vi "Create gplugindata payload.vi"(8 "error in":errorcluster, 9 "Library name with version":string, 10 "Relative Path":string, 11 "Display Name":string) -> (0 "error out":errorcluster, 3 "gplugindata":string)   [LabVIEW 2021, in "CIF Build Actions.lvlib"]
uses:
  CIF Build Actions.lvlib
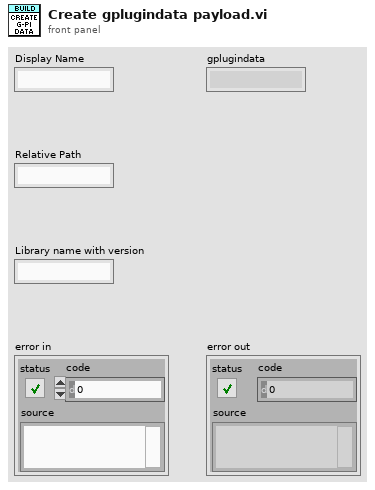
[diagram p1: front panel]
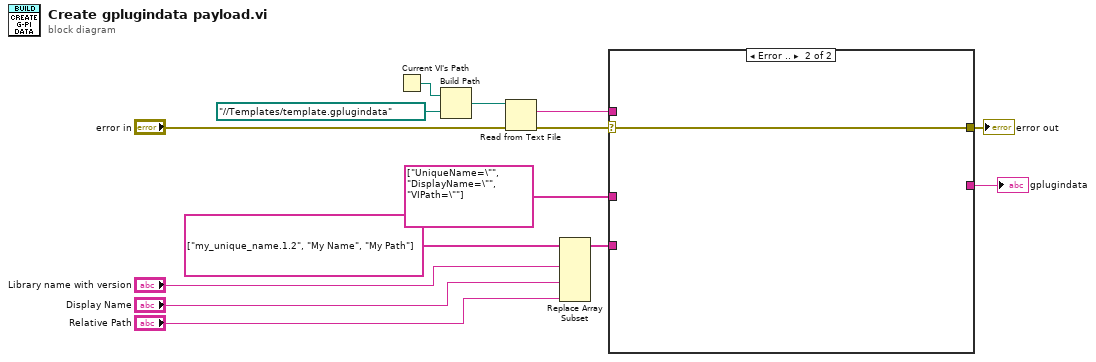
[diagram p0: block diagram]
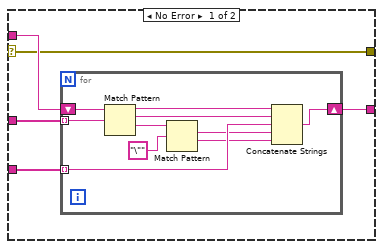
[diagram p2: hidden frame]
diagram:
  n1 = Current VI's Path() -> (path=w6:path)
  n2 = Build Path(base path=w6, name or relative path=path "../../Templates/template.gplugindata") -> (appended path=w5:path)
  n3 = Read from Text File(file (use dialog)=w5, error in="error in") -> (text=w7:string, error out=w2:errorcluster)  [unwired: 2 in, 2 out]
  n4 = Replace Array Subset(array=string[] ["my_unique_name.1.2", "My Name", "My Path"], new element #1="Library name with version", new element #2="Display Name", new element #3="Relative Path") -> (w10:string[])  [unwired: 3 in]
  n5 = case shown="Error .." w2 {
    selector: w2 -> [w15 w30]
    tunnel: [w19 _] -> w11
    tunnel: w10 -> [w18 _]
    tunnel: string[] ["UniqueName=\"", "DisplayName=\"", "VIPath=\""] -> [w17 _]
    tunnel: w7 -> [w16 _]
    tunnel: [w15 w30] -> w1
    frame No Error {
      n6 = for {
        tunnel: w18 -> [w23] mode=indexing
        tunnel: w17 -> [w28] mode=indexing
        shift-right: [w20] -> w19
        shift-left: w16 -> [w29]
        n7 = Match Pattern(string=w29, regular expression=w28) -> (before substring=w25:string, match substring=w24:string, after substring=w27:string)  [unwired: 1 in, 1 out]
        n8 = Match Pattern(string=w27, regular expression="\"") -> (match substring=w22:string, after substring=w21:string)  [unwired: 1 in, 2 out]
        n9 = Concatenate Strings(w25, w24, w23, w22, w21) -> (w20:string)
      }
    }
    frame Error {
    }
  }
  "gplugindata" <- w11
  "error out" <- w1
